vi "ApplicationGlobal.vi"() -> ()   [LabVIEW 2016]
uses:
  tools/Windows/Windows.ExitAction.ctl
panel:
  out "Runtime 2":bool
  in  "ImagesPath":path=path "D:/Maszup/WABCO/SVN/LaserMarkingStation/SOFTWARE/logs/results/images"
  out "Stats.Prog%":dbl format="%.3f"
  out "Station2":bool
  in  "TotalCounter":u32
  in  "StationNo":i32
  out "DMCConfig.Unlock":bool
  out "GuiRef.Stats":refnum<vi>
  out "GuiRef.DMCConfig":refnum<vi>
  out "Runtime":bool
  out "AppLaunched":bool
  out "GuiRef.Wait":refnum<vi>
  out "ManualView":bool
  out "Unlock":bool
  in  "font colors":u32[](array[colorbox])=[0, 0, 0, 0, 0, 0, 0, 16777226, 0, 0]
  in  "status colors":u32[](array[colorbox])=[16777226, 16775210, 16759552, 13816530, 7864153, 16744576, 8454143, 16711680, 16744640, 16744640]
  out "GuiRef.Results":refnum<vi>
  out "UnconfirmedError":bool
  out "Simulator":bool
  out "GuiRef.Base":refnum<vi>
  out "GuiRef.ChangeOver":refnum<vi>
  out "GuiRef.Daq":refnum<vi>
  out "GuiRef.Logs":refnum<vi>
  out "GuiRef.TestSteps":refnum<vi>
  in  "PlatesPath":path=path "D:/Maszup/WABCO/SVN/LaserMarkingStation/SOFTWARE/settings/plates"
  in  "EventPath":path=path "D:/Maszup/WABCO/SVN/LaserMarkingStation/SOFTWARE/logs/events"
  in  "ResultPath":path=path "D:/Maszup/WABCO/SVN/LaserMarkingStation/SOFTWARE/logs/results"
  out "AppDate":string
  in  "Status":string
  in  "ExitAction":T1=enum."Shut Down PC"
  out "AppName":string
  out "Changelog":string
  out "AppVer":string
  out "Quitting":bool
  in  "LogPath":path=path "D:/Maszup/WABCO/SVN/LaserMarkingStation/SOFTWARE/logs"
  in  "SettingsPath":path=path "D:/Maszup/WABCO/SVN/LaserMarkingStation/SOFTWARE/settings"
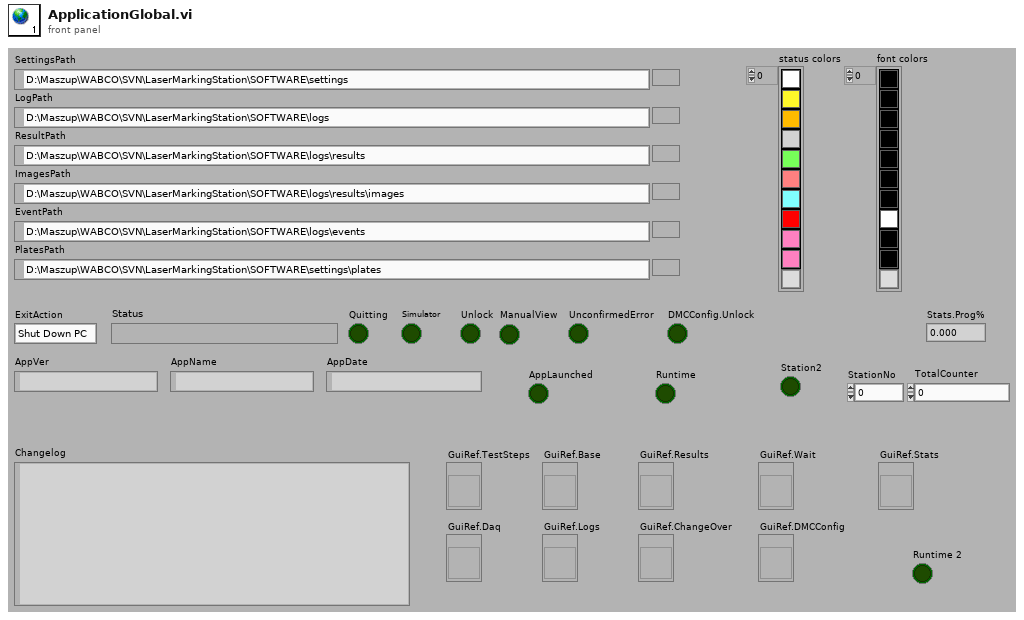
[diagram p1: front panel]
types:
  T1 = typedef "Windows.ExitAction.ctl" = enum16{"Log off from PC", "Shut Down PC", "Reboot PC", "Close Program"}
diagram:
